vi "ep_Check Nameplate (Torque).vi"(8 "error in (no error)":errorcluster, 10 "motor information":T2, 11 "nominal frequency":enum16{"50 Hz", "60 Hz"}(ring)) -> (0 "error out":errorcluster, 3 "information":T1)   [LabVIEW 2014, in "NI_EP_Motor Monitoring.lvlib"]
uses:
  <vilib>/addons/Electrical Power/Motor Monitoring/NI_EP_Motor Monitoring.lvlib
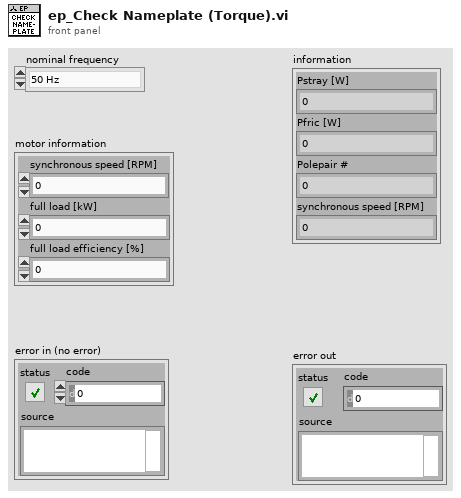
[diagram p1: front panel]
types:
  T1 = cluster{"Pstray [W]":dbl, "Pfric [W]":dbl, "Polepair #":i32, "synchronous speed [RPM]":dbl}
  T2 = cluster{"synchronous speed [RPM]":dbl, "full load [kW]":dbl, "full load efficiency [%]":dbl}
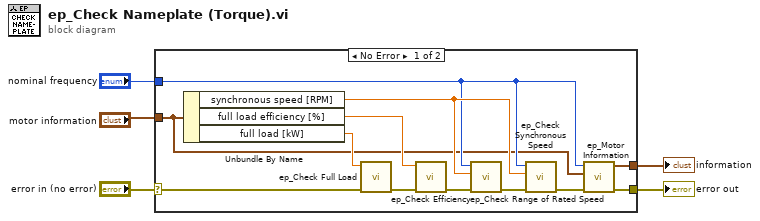
[diagram p0: block diagram]
diagram:
  n1 = case shown="No Error" "error in (no error)" {
    selector: "error in (no error)" -> [w8 w18]
    tunnel: [w12 w18] -> w4
    tunnel: "nominal frequency" -> [w11 _]
    tunnel: "motor information" -> [w10 _]
    tunnel: [w9 _] -> w1
    frame No Error {
      n2 = Unbundle By Name(w10) -> ("synchronous speed [RPM]"=w17:dbl, "full load efficiency [%]"=w15:dbl, "full load [kW]"=w16:dbl)
      n3 = call <vilib>:"ep_Check Full Load.vi"("error in (no error)"=w8, "full load [W]"=w16) -> ("error out"=w7:errorcluster)  [unwired: 9 in]
      n4 = call <vilib>:"ep_Check Efficiency.vi"("error in (no error)"=w7, "efficiency [%]"=w15) -> ("error out"=w6:errorcluster)  [unwired: 9 in]
      n5 = call <vilib>:"ep_Check Range of Rated Speed.vi"("error in (no error)"=w6, "speed [RPM]"=w17, "nominal frequency"=w11) -> ("error out"=w14:errorcluster)  [unwired: 8 in]
      n6 = call <vilib>:"ep_Check Synchronous Speed.vi"("error in (no error)"=w14, "synchronous speed [RPM]"=w17, "nominal frequency"=w11) -> ("error out"=w13:errorcluster)  [unwired: 8 in]
      n7 = call <vilib>:"ep_Motor Information.vi"("error in (no error)"=w13, "motor information"=w10, "nominal frequency"=w11) -> ("error out"=w12:errorcluster, "information"=w9:T1)  [unwired: 7 in]
    }
    frame Error {
    }
  }
  "error out" <- w4
  "information" <- w1
